vi "midterm-4.vi"() -> ()   [LabVIEW 2024]
uses:
  <userlib>/ME121-25-main/ME121-25-main/LabVIEW/SerialVIs/subs/portX.xctl
panel:
  in  "Initial Postion":cluster{"x-position":dbl, "y-position":dbl}={"x-position"=0.0, "y-position"=162.5} {"y-position" scale=0.0..162.5; "x-position" scale=0.0..162.5}
  out "Final and Initial Position sent to motors":string="main(-85,66,18,-112,57,56)\r\n"
  in  "STOP":bool
  out "Arms":picture
  in  "?":refnum<visa-resource-name>(xcontrol)="ASRL15"
  out "2D Picture":picture
  out "Ending Position":cluster{"X":i32, "Y":i32}
  in  "stop":bool
  # "ME-121-3DOF- MIDTERM"
  # "1) Choose Port"
  # "VI Overview\n\nThis LabVIEW VI controls a 3DoF robotic arm with two links and a chair attached to the end effector. \nThe objective is to move the arm while keeping the chair level to prevent a seated LEGO figure from falling.\nFeatures:\n\n    - Select initial and final positions\n    - Perform inverse kinematics (IK) to compute joint angles\n    - Communicate with a microcontroller to send movement commands\n    - Display a 2D visualization of the arm and its reachable workspace"
  # "Angle 3"
  # "Choose arm length"
  # "User Guide:\n\n    1- Connect to the microcontroller via the port on the right.\n    2 -Select initial and final positions.\n    3 - Click Run:\n       - If the position is within range, a 2D visualization appears, and the user is prompted to execute the                                            \n          movement.\n       -  If out of range, the user is asked to select a valid position.\n\nLet me know if you need further refinements!"
  # "Angle 2"
  # "Angle 1"
  # "3) Click to choose position to go to"
  # "2) Choose Initial Position"
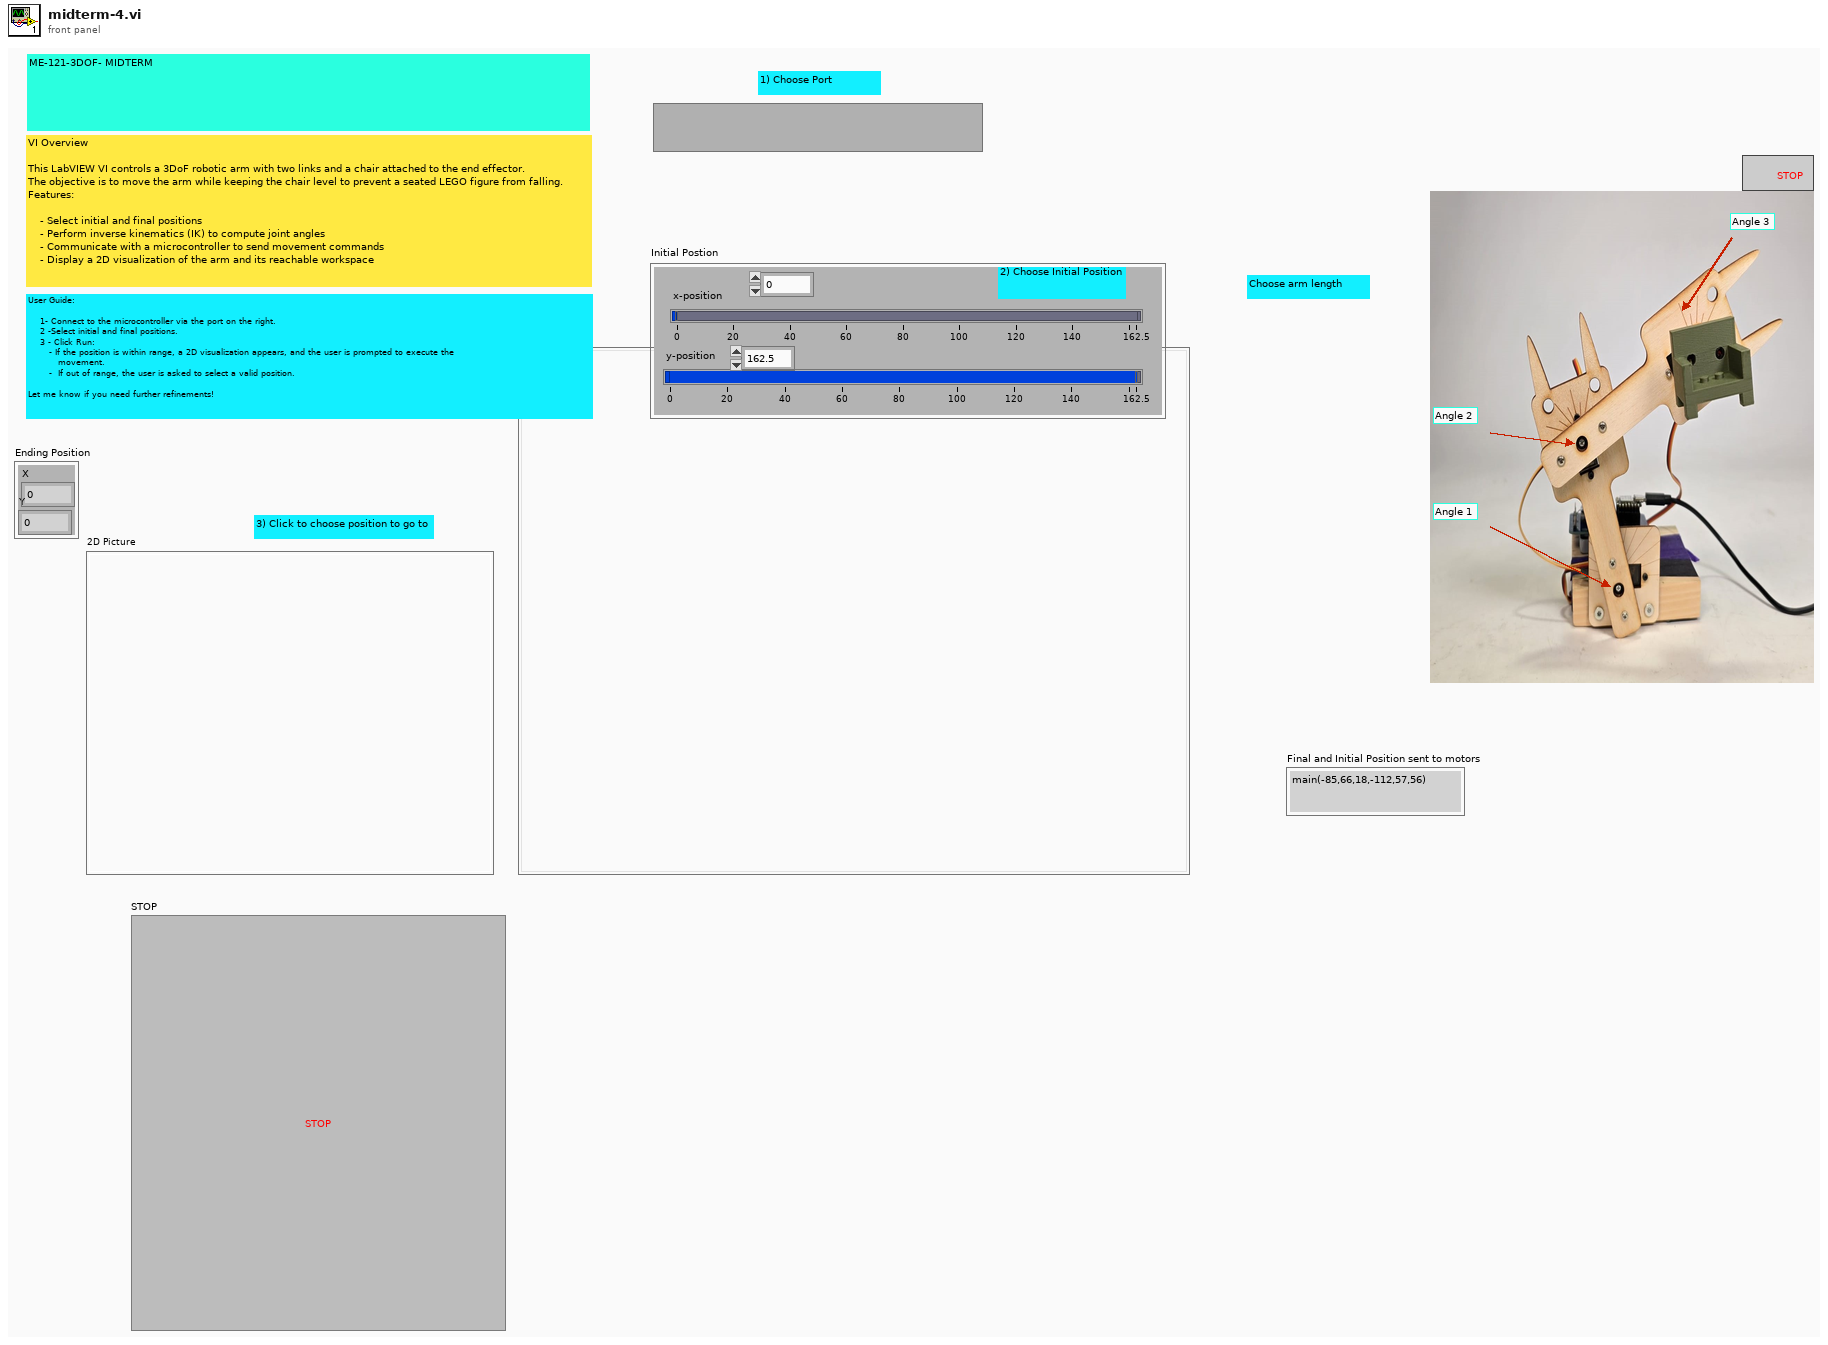
[diagram p1: front panel]
types:
  T1 = cluster{"Width":u16, "Style":enum32{"Solid", "Dash", "Dot", "DashDot", "DashDotDot"}}
  T2 = typedef "lveventtype.ctl" = enum32{"Null", "Timeout", "Annotation Menu Selection", "Annotation Menu Selection?", "App Instance Close", "App Instance Close?", "Autoscale Range Change", "Bookmark Info Change", "Cell Edit", "Cell Edit?", "Cursor Grab", "Cursor Grab?", "Cursor Menu Selection", "Cursor Menu Selection?", "Cursor Move", "Cursor Release", "Data Change", "Direction Change", "Display State Change", "Drag Ended", "Drag Enter", "Drag Leave", "Drag Over", "Drag Source Update", "Drag Starting", "Drag Starting?", "Drop", "Exec State Change", "Key Down", "Key Down?", "Key Repeat", "Key Repeat?", "Key Up", "Listbox Double Click", "Menu Activation?", "Menu Selection (App)", "Menu Selection? (App)", "Menu Selection (User)", "Mouse Down", "Mouse Down?", "Mouse Enter", "Mouse Leave", "Mouse Move", "Mouse Up", "Mouse Wheel", "NI Security User Change (App)", "Pane Size", "Panel Close", "Panel Close?", "Panel Resize", "Plot Attribute Change", "Scale Range Change", "Shortcut Menu Activation?", "Shortcut Menu Selection (App)", "Shortcut Menu Selection? (App)", "Shortcut Menu Selection (User)", "Tree Double Click", "Tree Drag", "Tree Drag?", "Tree Drop", "Tree Drop?", "Tree Item Close", "Tree Item Close?", "Tree Item Open", "Tree Item Open?", "User Event", "Value Change"}
  T3 = typedef "LVMouseTypeDef.ctl" = cluster{"Mouse Position":cluster{"X":i32, "Y":i32}, "Mouse Modifiers":cluster{"Button Down":bool, "Shift Mod":bool, "Menu Mod":bool, "Option Mod":bool}}
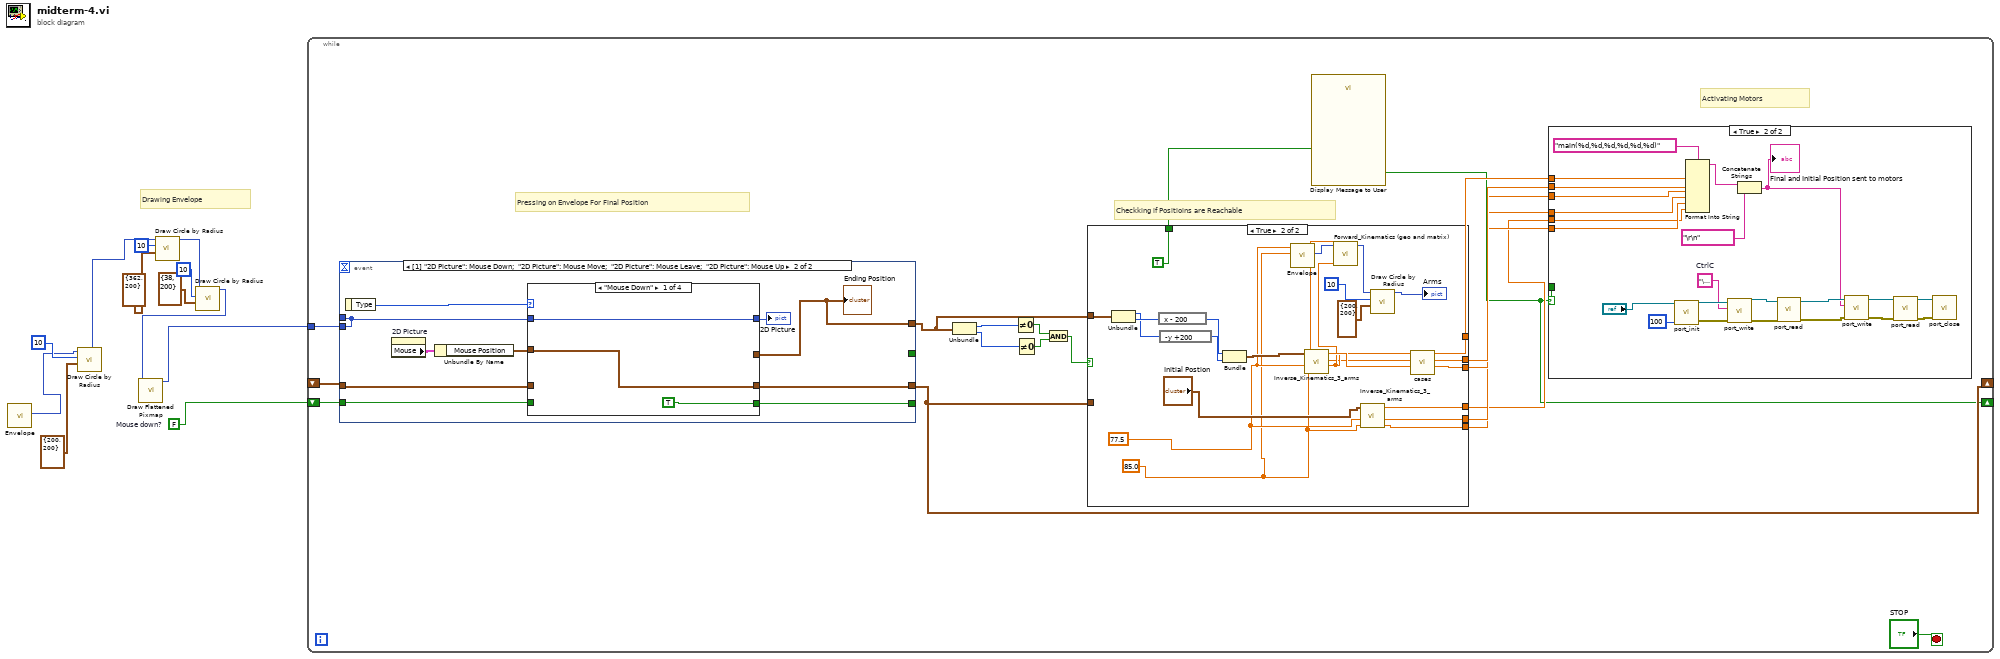
[diagram p0: block diagram]
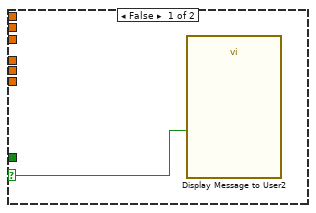
[diagram p2: hidden frame]
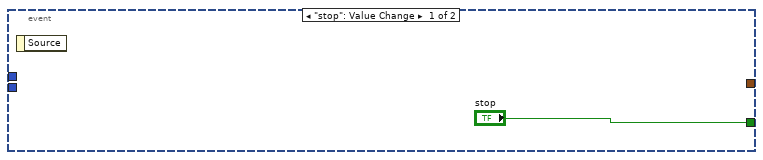
[diagram p4: hidden frame]
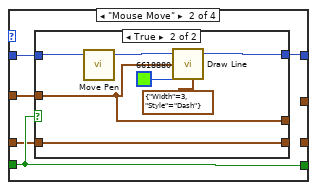
[diagram p5: hidden frame]
diagram:
  w11 = FALSE  # Mouse down?
  # "Drawing Envelope"
  n1 = call "Envelope.vi"() -> ("new picture"=w9:picture)  [unwired: 11 in]
  n2 = call <vilib>:"Draw Circle by Radius.vi"("pixel center"=cluster{"horizontal":i16, "vertical":i16} {"horizontal"=200, "vertical"=200}, "radius"=i16 10, "picture"=w9) -> ("new picture"=w7:picture)  [unwired: 8 in]
  n3 = call <vilib>:"Draw Circle by Radius.vi"("pixel center"=cluster{"horizontal":i16, "vertical":i16} {"horizontal"=362, "vertical"=200}, "radius"=i16 10, "picture"=w7) -> ("new picture"=w6:picture)  [unwired: 8 in]
  n4 = call <vilib>:"Draw Circle by Radius.vi"("pixel center"=cluster{"horizontal":i16, "vertical":i16} {"horizontal"=38, "vertical"=200}, "radius"=i16 10, "picture"=w6) -> ("new picture"=w1:picture)  [unwired: 8 in]
  n5 = call <vilib>:"Draw Flattened Pixmap.vi"("picture"=w1) -> ("new picture"=w12:picture)  [unwired: 8 in]
  n6 = while {
    tunnel: w12 -> [w31]
    shift-right: [w14] -> _
    shift-left: _ -> [w29]
    shift-right: [w13] -> _
    shift-left: w11 -> [w30]
    stop <- "STOP" stop-if-true
    # "Checkking if Positioins are Reachable"
    # "Activating Motors"
    # "Pressing on Envelope For Final Position"
    n7 = event shown="[1] \"2D Picture\": Mouse Down;  \"2D Picture\": Mouse Move;  \"2D Picture\": Mouse Leave;  \"2D Picture\": Mouse Up" {
      selector: _ -> [_ _]
      dyn-events: _ -> [_ _]
      timeout: _ -> [_ _]
      tunnel: ["stop" _] -> _
      tunnel: [_ w82] -> _
      tunnel: [_ w91] -> _
      tunnel: w30 -> [_ w87]
      tunnel: [_ w86] -> w14
      tunnel: w29 -> [_ w85]
      tunnel: [_ w83] -> w24
      tunnel: w31 -> [_ w82]
      event "stop": Value Change {
        n8 = event-data() -> ()  [unwired: 1 in, 1 out]
      }
      event "2D Picture": Mouse Down; "2D Picture": Mouse Move; "2D Picture": Mouse Leave; "2D Picture": Mouse Up {
        n9 = event-data() -> ("Type"=w90:T2)  [unwired: 1 in]
        n10 = property on="2D Picture" class="Pict"() -> ("Mouse"=w88:T3)  [unwired: 2 in, 2 out]
        n11 = Unbundle By Name(w88) -> ("Mouse Position"=w84:cluster{"X":i32, "Y":i32})
        n12 = case shown="\"Mouse Down\"" w90 {
          tunnel: [TRUE ("fill?(F)") w96 _ _] -> w91
          tunnel: w82 -> [w92 w98 w109 w110]
          tunnel: [w92 w99 w109 w110] -> w89
          tunnel: w84 -> [w93 w97 _ w111]
          tunnel: w87 -> [_ w96 _ _]
          tunnel: [w93 _ _ _] -> w86
          tunnel: w85 -> [_ w95 _ _]
          tunnel: [_ _ _ w111] -> w83
          frame "Mouse Down" {
          }
          frame "Mouse Move" {
            n13 = case shown="True" w96 {
              tunnel: [w101 w108] -> w99
              tunnel: w98 -> [w101 w106]
              tunnel: w97 -> [_ w102]
              tunnel: [w100 w104] -> _
              tunnel: w95 -> [w100 w104]
              tunnel: [_ w102] -> _
              frame False {
                # "Mouse is up, ignore"
              }
              frame True {
                n14 = call <vilib>:"Move Pen.vi"("picture"=w106) -> ("new picture"=w105:picture)  [unwired: 4 in]
                n15 = call <vilib>:"Draw Line.vi"("picture"=w105, "end point"=w102, "color(black)"=u32 6618880, "pen"=T1 {"Width"=3, "Style"=enum."Dash"}) -> ("new picture"=w108:picture)  [unwired: 5 in]
              }
            }
          }
          frame Default {
            # "reset on mouse up, mouse leave, etc."
          }
          frame "Mouse Up" {
          }
        }
        "2D Picture" <- w89
        "Ending Position" <- w83
      }
    }
    n16 = Unbundle(w24) -> ("X"=w28:i32, "Y"=w27:i32)
    n17 = Not Equal To 0?(x=w28) -> (x != 0?=w25:bool)
    n18 = Not Equal To 0?(x=w27) -> (x != 0?=w26:bool)
    n19 = And(x=w25, y=w26) -> (x .and. y?=w23:bool)
    n20 = case shown="True" w23 {
      tunnel: w24 -> [_ w76]
      tunnel: [_ w75] -> w22
      tunnel: [_ w74] -> w21
      tunnel: [_ w73] -> w20
      tunnel: [_ w72] -> w19
      tunnel: [_ w71] -> w18
      tunnel: [_ w70] -> w17
      tunnel: [_ TRUE] -> w15
      tunnel: w14 -> [_ _]
      frame False {
      }
      frame True {
        w57 = 85.0 ("L 1")
        w58 = 77.5 ("L 1")
        n21 = Unbundle(w76) -> ("X"=w61:i32, "Y"=w60:i32)
        n22 = expression code="x - 200"(w61) -> (w79:i32)
        n23 = expression code="-y +200"(w60) -> (w78:i32)
        n24 = Bundle("X"=w79, "Y"=w78) -> (w77:cluster{"X":i32, "Y":i32})  [unwired: 1 in]
        n25 = call "Envelope.vi"("L 2"=w57, "L 1"=w58) -> ("new picture"=w66:picture)  [unwired: 9 in]
        n26 = call "Inverse_Kinematics_3_arms.vi"("L 2"=w57, "L 1"=w58, "end effector"=w77) -> ("Angle 2"=w62:dbl, "Angle1"=w63:dbl, "Angle 3"=w80:dbl)  [unwired: 6 in]
        n27 = call "Forward_Kinematics (geo and matrix).vi"("q2"=w62, "q1"=w63, "new picture"=w66) -> ("2D Picture"=w67:picture)  [unwired: 6 in, 2 out]
        n28 = call "Inverse_Kinematics_3_arms.vi"("L 2"=w57, "L 1"=w58, "end effector"="Initial Postion") -> ("Angle 2"=w71:dbl, "Angle1"=w72:dbl, "Angle 3"=w70:dbl)  [unwired: 6 in]
        n29 = call <vilib>:"Draw Circle by Radius.vi"("pixel center"=cluster{"horizontal":i16, "vertical":i16} {"horizontal"=200, "vertical"=200}, "radius"=i16 10, "picture"=w67) -> ("new picture"=→"Arms":picture)  [unwired: 8 in]
        n30 = call "cases.vi"("q 3"=w80, "q 2"=w62, "q 1"=w63) -> ("q3"=w73:dbl, "q2"=w74:dbl, "q1"=w75:dbl)  [unwired: 6 in]
      }
    }
    n31 = call "Display Message to User"("Enable"=w15) -> ("OK"=w13:bool)  [unwired: 9 in, 1 out]
    n32 = case shown="True" w13 {
      selector: w13 -> [w32 w37]
      tunnel: w22 -> [_ w43]
      tunnel: w21 -> [_ w42]
      tunnel: w20 -> [_ w41]
      tunnel: w19 -> [_ w40]
      tunnel: w18 -> [_ w39]
      tunnel: w17 -> [_ w38]
      tunnel: [_ w37] -> _
      frame False {
        n33 = call "Display Message to User2"("Enable"=w32) -> ()  [unwired: 9 in, 2 out]
      }
      frame True {
        w48 = "\u0003"  # CtrlC
        n34 = call <userlib>:"port_init.vi"("Timeout (ms)"=u32 100, "VISA Refnum in"="?") -> ("error out"=w53:errorcluster, "VISA Refnum out"=w54:refnum<visa-resource-name>)  [unwired: 8 in]
        n35 = Format Into String(format string="main(%d,%d,%d,%d,%d,%d)", w43, w42, w41, w40, w39, w38) -> (resulting string=w35:string)  [unwired: 2 in, 1 out]
        n36 = call <userlib>:"port_write.vi"("error in (no error)"=w53, "write buffer"=w48, "VISA Refnum in"=w54) -> ("error out"=w51:errorcluster, "VISA Refnum out"=w52:refnum<visa-resource-name>)  [unwired: 7 in]
        n37 = Concatenate Strings(w35, "\r\n") -> (w33:string)
        "Final and Initial Position sent to motors" <- w33
        n38 = call <userlib>:"port_read.vi"("error in (no error)"=w51, "VISA Refnum in"=w52) -> ("error out"=w47:errorcluster, "VISA Refnum out"=w46:refnum<visa-resource-name>)  [unwired: 7 in, 1 out]
        n39 = call <userlib>:"port_write.vi"("error in (no error)"=w47, "write buffer"=w33, "VISA Refnum in"=w46) -> ("error out"=w56:errorcluster, "VISA Refnum out"=w55:refnum<visa-resource-name>)  [unwired: 7 in]
        n40 = call <userlib>:"port_read.vi"("error in (no error)"=w56, "VISA Refnum in"=w55) -> ("error out"=w45:errorcluster, "VISA Refnum out"=w44:refnum<visa-resource-name>)  [unwired: 7 in, 1 out]
        n41 = call <userlib>:"port_close.vi"("error in (no error)"=w45, "VISA Refnum in"=w44) -> ()  [unwired: 10 in]
      }
    }
  }
